vi "Configure Relative Calculation.vi"(0 "VISA resource name":refnum<visa-resource-name>, 1 "Enable Rel (F: Disable)":bool, 2 "Rel Value (0)":dbl, 5 "Use Input Signal As Rel Value (F: Disable)":bool, 11 "error in (no error)":errorcluster) -> (4 "VISA resource name out":refnum<visa-resource-name>, 15 "error out":errorcluster)   [LabVIEW 2016, in "Keithley 6517.lvlib"]
doc: "Configures Baseline (Relative) Value settings.\n\nRelative (Rel) nulls an offset or subtracts a baseline reading from present and future readings. When a Rel value is established, subsequent readings will be the difference between the actual input and the Rel value.\n\n<B>Displayed (Rel'ed) Reading = Actual Input - Rel Value</B>\n\n<B>Note:</B>\n(1)Note that function changes disables Rel.\n(2)This VI is ONLY compatible with <B>model 6514</B>. Running this VI with any other model will result in an error."
uses:
  <instrlib>/Keithley 6517/Keithley 6517.lvlib
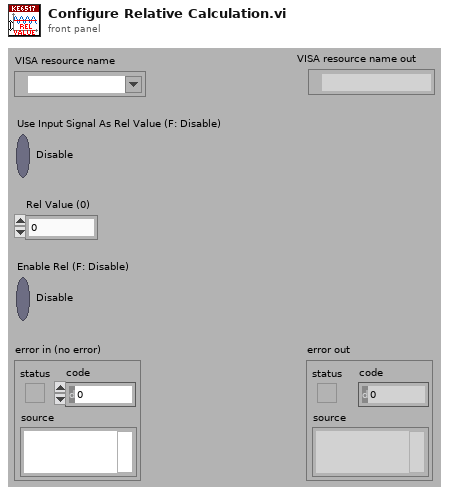
[diagram p1: front panel]
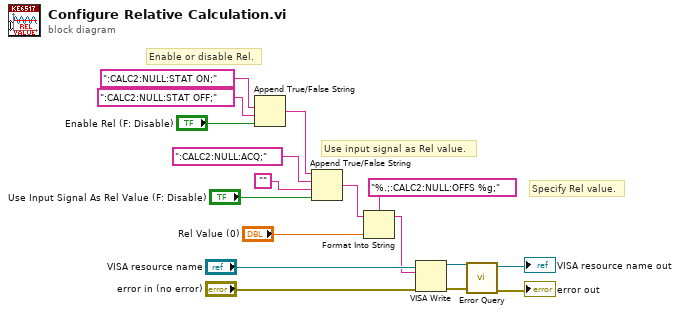
[diagram p0: block diagram]
diagram:
  # "Specify Rel value."
  # "Use input signal as Rel value."
  # "Enable or disable Rel."
  n1 = Append True/False String(1:"Enable Rel (F: Disable)", 2:":CALC2:NULL:STAT OFF;" ("false string"), 3:":CALC2:NULL:STAT ON;" ("true string")) -> (0:w6:string)  [unwired: 1 in]
  n2 = Append True/False String(1:"Use Input Signal As Rel Value (F: Disable)", 2:"", 3:":CALC2:NULL:ACQ;" ("true string"), 4:w6) -> (0:w5:string)
  n3 = Format Into String(format string="%.;:CALC2:NULL:OFFS %g;", initial string=w5, "Rel Value (0)") -> (resulting string=w2:string)  [unwired: 1 in, 1 out]
  n4 = VISA Write(VISA resource name="VISA resource name", write buffer=w2, error in (no error)="error in (no error)") -> (VISA resource name out=w9:refnum<visa-resource-name>, error out=w10:errorcluster)  [unwired: 1 out]
  n5 = call <instrlib>:"Error Query.vi"("error in (no error)"=w10, "VISA resource name"=w9) -> ("error out"=→"error out":errorcluster, "VISA resource name out"=→"VISA resource name out":refnum<visa-resource-name>)  [unwired: 6 in, 2 out]
